vi "Disconnect.vi"(8 "error in":errorcluster, 11 "36234A in":refnum<class "36234A.lvclass">) -> (0 "error out":errorcluster, 3 "36234A out":refnum<class "36234A.lvclass">)   [LabVIEW 2019, in "36234A.lvlib" / "36234A.lvclass"]
doc: "This disconnect routine is a must override from the Instrument Class\nChildren Classes are responsible for handling the override, but the parent class is an intermediary and must contain the override functions to maintain the rules for the method."
uses:
  Library/36234A.lvclass
  Library/36234A.lvclass/36234A.ctl
  builds/Instruments/PowerSupply.lvlibp/Library/PowerSupply.lvclass
  <instrlib>/Keysight E36000 Series/Keysight E36000 Series.lvlib
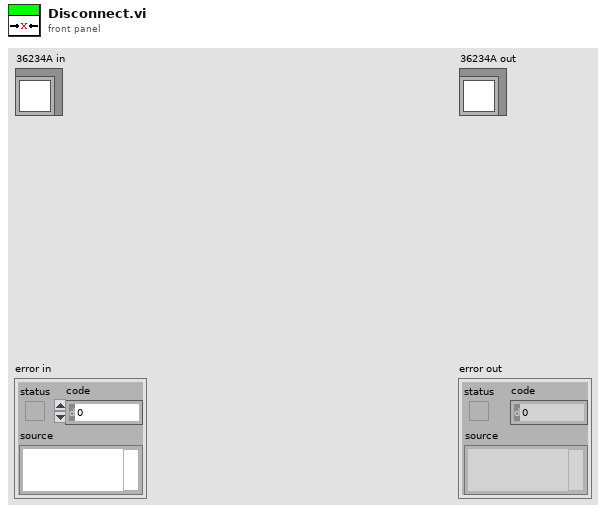
[diagram p1: front panel]
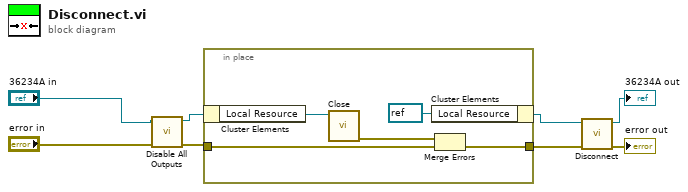
[diagram p0: block diagram]
diagram:
  n1 = call "Disable All Outputs.vi"("error in"="error in", "36234A in"="36234A in") -> ("error out"=w1:errorcluster, "36234A out"=w3:refnum<class "36234A.lvclass">)  [unwired: 8 in]
  n2 = in-place {
    in-place-border: w1 -> [w10]
    in-place-border: [w9] -> w5
    n3 = in-place-cluster #1(w3) -> ("Local Resource"=w12:refnum<visa-resource-name>)
    n4 = call <instrlib>:"Close.vi"("VISA resource name"=w12) -> ("error out"=w11:errorcluster)  [unwired: 10 in]
    n5 = in-place-cluster #1("Local Resource"=refnum<visa-resource-name> refnum) -> (w6:refnum<class "36234A.lvclass">)
    n6 = Merge Errors(w11, w10) -> (w9:errorcluster)
  }
  n7 = call-parent "Disconnect.vi"("error in"=w5, "PowerSupply in"=w6) -> ("error out"=→"error out":errorcluster, "PowerSupply out"=→"36234A out":refnum<class "36234A.lvclass">)  [unwired: 8 in]
